vi "WILT Array 2D RW str.vi"(0 "file path (dialog if empty)":path=path "c:/data/text.csv", 5 "Write/Read":T1(ring), 7 "2D Sample Array In":string[][](array[string])=[["1", "2\n2\n2-3", "3"], ["a", "b", "c-1\nc-2\nc-3"]], 9 "1D Sample Append Array":string[](array[string])=["1", "2\n2\n2-3", "3"]) -> (8 "Read all rows":string[][](array[string]))   [LabVIEW 2016]
uses:
  Globals/Globals Wilt.vi
  <vilib>/Utility/file.llb/Read From Spreadsheet File (string).vi
panel:
  out "number of replacements":i32
  out "Parsed  Elements":i32
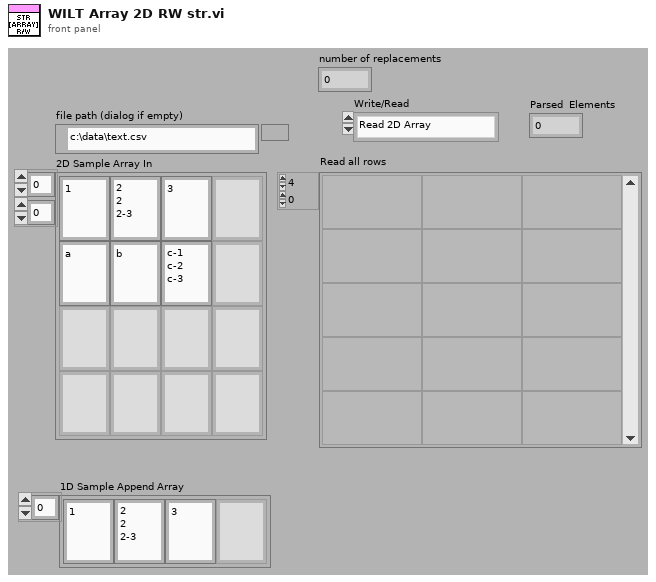
[diagram p1: front panel]
types:
  T1 = enum16{"Read 2D Array", "Write 2D Array", "Write/Append 1D Array"}
  T2 = enum16{"open", "replace", "create", "open or create", "replace or create", "replace or create with confirmation"}
  T3 = enum16{"deny read/write", "deny write-only", "deny none"}
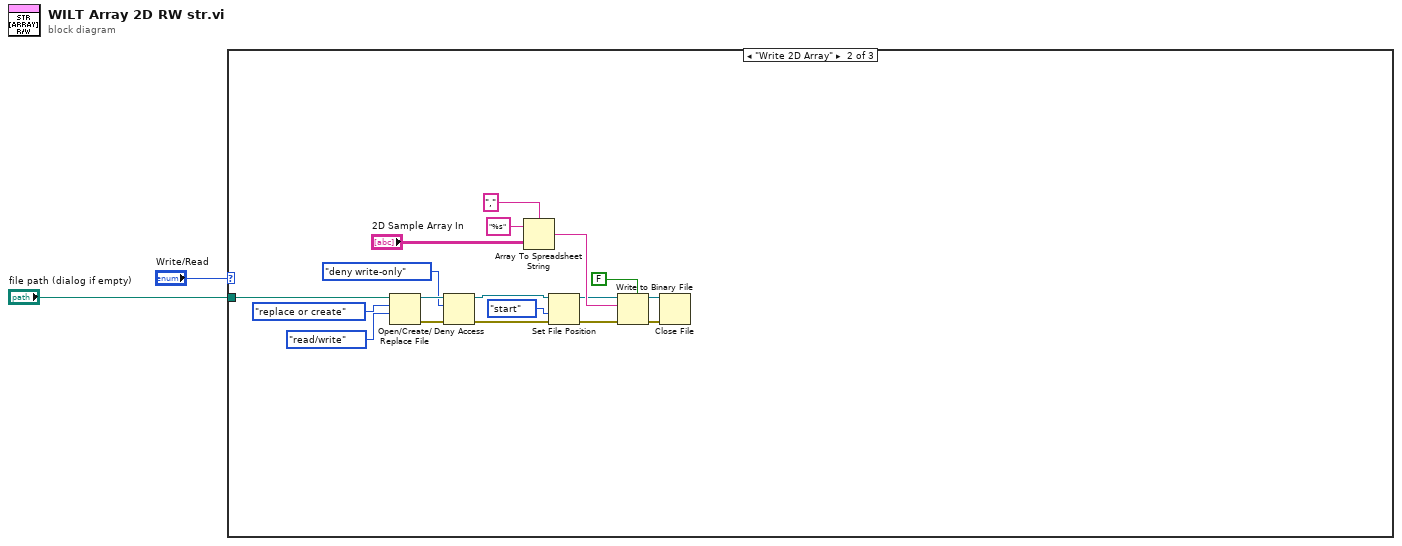
[diagram p0: block diagram]
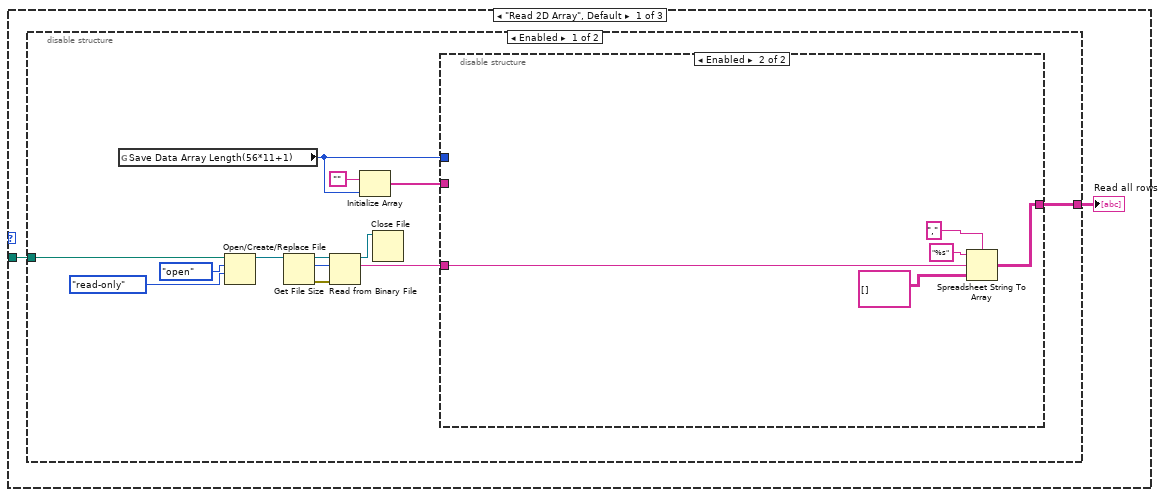
[diagram p2: hidden frame]
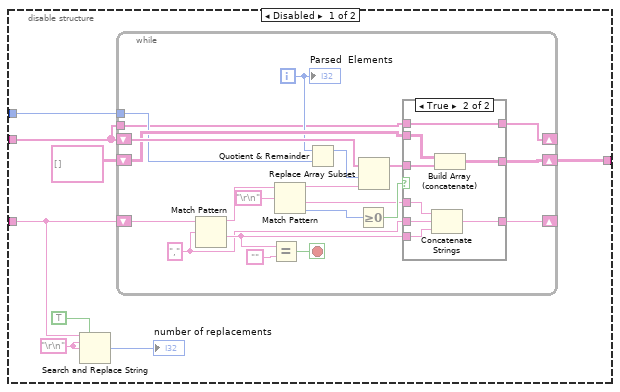
[diagram p3: hidden frame]
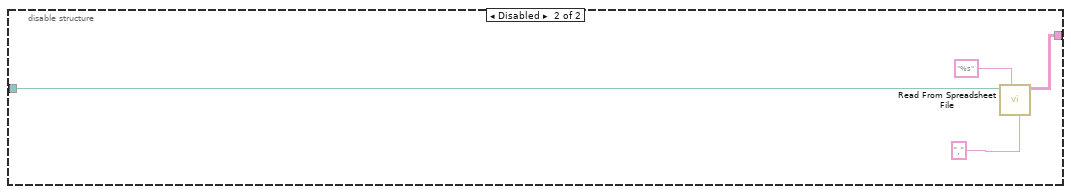
[diagram p5: hidden frame]
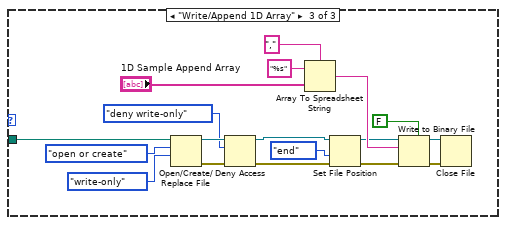
[diagram p6: hidden frame]
diagram:
  n1 = case shown="\"Write 2D Array\"" "Write/Read" {
    tunnel: "file path (dialog if empty)" -> [w3 w78 w96]
    frame "Read 2D Array", Default {
      n2 = disable-structure shown="Enabled" {
        disable-tunnel: [w17 w63] -> w4
        disable-tunnel: w3 -> [w16 w66]
        frame Enabled {
          n3 = global read "Globals Wilt.vi" "Save Data Array Length(56*11+1)"() -> (w7:i32)
          n4 = Open/Create/Replace File(file path (use dialog)=w16, operation (0:open)=T2."open", access (0:read/write)=enum16{"read/write", "read-only", "write-only"}."read-only") -> (refnum out=w12:refnum<file>)  [unwired: 3 in, 2 out]
          n5 = Get File Size(file=w12) -> (refnum out=w11:refnum<file>, size (in bytes)=w9:i64, 0:w10:errorcluster)  [unwired: 1 in]
          n6 = Read from Binary File(8:w10, 10:w9, 11:w11) -> (2:w5:string, 3:w13:refnum<file>)  [unwired: 3 in, 2 out]
          n7 = Initialize Array("", w7) -> (w6:string[])
          n8 = Close File(refnum=w13) -> ()  [unwired: 1 in, 2 out]
          n9 = disable-structure shown="Enabled" {
            disable-tunnel: [w24 w60] -> w17
            disable-tunnel: w5 -> [w21 w62]
            disable-tunnel: w7 -> [w23 _]
            disable-tunnel: w6 -> [w22 _]
            frame Disabled {
              w20 = "\r\n"
              n10 = Search and Replace String(replace all?=TRUE ("replace all? (F)"), input string=w21, search string=w20, replace string=w20) -> (number of replacements=→"number of replacements":i32)  [unwired: 4 in, 3 out]
              n11 = while {
                shift-right: [w38] -> _
                shift-left: w21 -> [w46]
                shift-right: [w33] -> _
                shift-left: w22 -> [w40]
                shift-right: [w35] -> w24
                shift-left: string[][] [] -> [w34]
                tunnel: w23 -> [w29]
                tunnel: w22 -> [w26]
                i -> [w30]
                stop <- w41 stop-if-true
                w31 = "," ("regular expression")
                n12 = Match Pattern(string=w46, regular expression=w31) -> (before substring=w45:string, after substring=w37:string)  [unwired: 1 in, 2 out]
                n13 = Equal?(x=w37, y="") -> (x = y?=w41:bool)
                n14 = Match Pattern(string=w45, regular expression="\r\n") -> (before substring=w28:string, after substring=w36:string, offset past match=w43:i32)  [unwired: 1 in, 1 out]
                n15 = Quotient & Remainder(x=w30, y=w29) -> (x-y*floor(x/y)=w27:i32)  [unwired: 1 out]
                n16 = Greater Or Equal To 0?(x=w43) -> (x >= 0?=w39:bool)
                n17 = Replace Array Subset(array=w40, new element=w28, index=w27) -> (w32:string[])
                n18 = case shown="True" w39 {
                  tunnel: [w49 w56] -> w38
                  tunnel: w37 -> [w49 w57]
                  tunnel: w36 -> [_ w52]
                  tunnel: [w48 w55] -> w35
                  tunnel: w34 -> [w48 w54]
                  tunnel: [w47 w51] -> w33
                  tunnel: w32 -> [w47 w50]
                  tunnel: w31 -> [_ w53]
                  tunnel: w26 -> [_ w51]
                  frame False {
                  }
                  frame True {
                    n19 = Concatenate Strings(w52, w53, w57) -> (w56:string)
                    n20 = Build Array (concatenate)(w54, w50) -> (w55:string[][])
                  }
                }
                "Parsed  Elements" <- w30
              }
            }
            frame Enabled {
              n21 = Spreadsheet String To Array(delimiter (Tab)=",", format string="%s", spreadsheet string=w62, array type (2D Dbl)=string[][] []) -> (array=w60:string[][])
            }
          }
        }
        frame Disabled {
          n22 = call-poly <vilib>:"Read From Spreadsheet File.vi"("delimiter (\\t)"="," ("delimiter (\\t)"), "format (%s)"="%s", "file path (dialog if empty)"=w66) -> ("all rows"=w63:string[][])  [unwired: 4 in, 4 out]
        }
      }
      "Read all rows" <- w4
    }
    frame "Write 2D Array" {
      n23 = Open/Create/Replace File(file path (use dialog)=w78, operation (0:open)=T2."replace or create", access (0:read/write)=enum16{"read/write", "read-only", "write-only"}."read/write") -> (refnum out=w75:refnum<file>, error out=w76:errorcluster)  [unwired: 3 in, 1 out]
      n24 = Deny Access(4:w76, 6:T3."deny write-only" ("deny mode (0:deny read/write)"), 7:w75) -> (0:w71:errorcluster, 3:w69:refnum<file>)
      n25 = Array To Spreadsheet String(delimiter (Tab)=",", array="2D Sample Array In", 3:"%s" ("format string")) -> (spreadsheet string=w81:string)
      n26 = Set File Position(refnum=w69, from (0:start)=enum16{"start", "end", "current"}."start", error in=w71) -> (refnum out=w68:refnum<file>, error out=w70:errorcluster)  [unwired: 1 in]
      n27 = Write to Binary File(file (use dialog)=w68, data=w81, error in=w70, 5:FALSE ("prepend array or string size? (T)")) -> (refnum out=w77:refnum<file>, error out=w73:errorcluster)  [unwired: 2 in, 1 out]
      n28 = Close File(refnum=w77, error in=w73) -> ()  [unwired: 2 out]
    }
    frame "Write/Append 1D Array" {
      n29 = Open/Create/Replace File(file path (use dialog)=w96, operation (0:open)=T2."open or create", access (0:read/write)=enum16{"read/write", "read-only", "write-only"}."write-only") -> (refnum out=w93:refnum<file>, error out=w94:errorcluster)  [unwired: 3 in, 1 out]
      n30 = Deny Access(4:w94, 6:T3."deny write-only" ("deny mode (0:deny read/write)"), 7:w93) -> (0:w89:errorcluster, 3:w87:refnum<file>)
      n31 = Array To Spreadsheet String(delimiter (Tab)=",", array="1D Sample Append Array", 3:"%s" ("format string")) -> (spreadsheet string=w99:string)
      n32 = Set File Position(refnum=w87, from (0:start)=enum16{"start", "end", "current"}."end", error in=w89) -> (refnum out=w86:refnum<file>, error out=w88:errorcluster)  [unwired: 1 in]
      n33 = Write to Binary File(file (use dialog)=w86, data=w99, error in=w88, 5:FALSE ("prepend array or string size? (T)")) -> (refnum out=w95:refnum<file>, error out=w91:errorcluster)  [unwired: 2 in, 1 out]
      n34 = Close File(refnum=w95, error in=w91) -> ()  [unwired: 2 out]
    }
  }
